vi "Output Enable Write Single.vi"(8 "error in":errorcluster, 9 "Channel Index":i32=1, 10 "Output Enable STS":dbl, 11 "Power Supply In":refnum<class "Power Supply.lvclass">) -> (0 "error out":errorcluster, 3 "Power Supply Out":refnum<class "Power Supply.lvclass">)   [LabVIEW 2023, in "Power Supply.lvclass"]
uses:
  Power Supply.lvclass
  Power Supply.lvclass/Power Supply.ctl
  Low Level Capabilities/Output Enable/Output Enable.lvclass
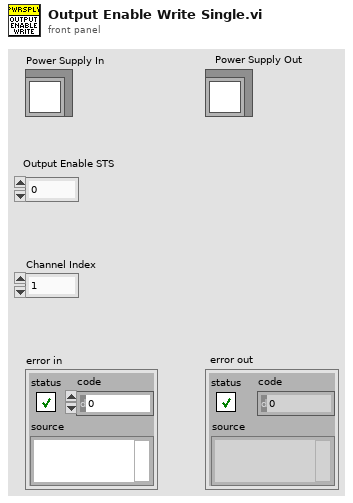
[diagram p1: front panel]
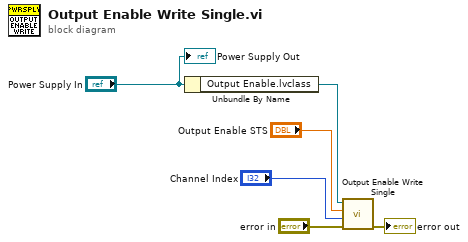
[diagram p0: block diagram]
diagram:
  n1 = Unbundle By Name("Power Supply In") -> ("Output Enable.lvclass"=w1:refnum<class "Output Enable.lvclass">)
  n2 = call-dynamic "Output Enable Write Single.vi"("error in"="error in", "Channel Index"="Channel Index", "Output Enable STS"="Output Enable STS", "Output Enable in"=w1) -> ("error out"=→"error out":errorcluster)  [unwired: 6 in, 1 out]
  "Power Supply Out" <- "Power Supply In"
